vi "Encrypt.vi"(8 "error in (no error)":errorcluster, 10 "Arguments":string[](array[string]), 11 "Encryption in":refnum<class "Encryption.lvclass">) -> (0 "error out":errorcluster, 2 "Encrypted Arguments":string[](array[string]), 3 "Encryption out":refnum<class "Encryption.lvclass">)   [LabVIEW 2019, in "TSC Event Logger.lvlib" / "Encryption.lvclass"]
uses:
  Encryption.lvclass
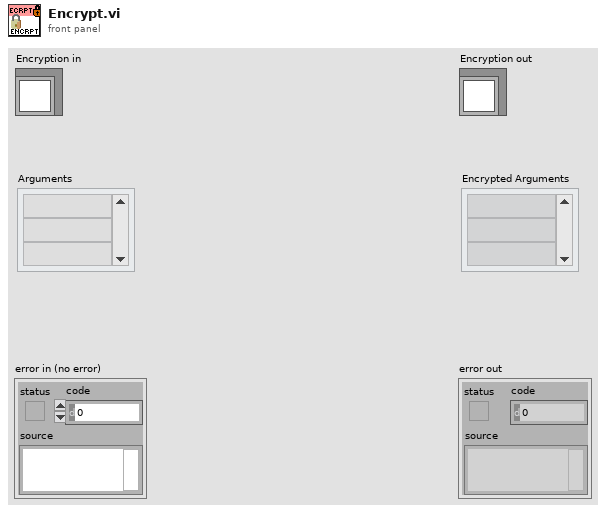
[diagram p1: front panel]
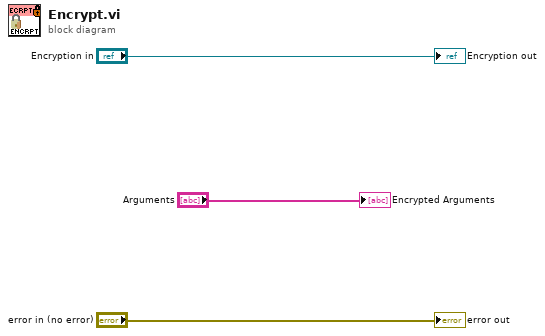
[diagram p0: block diagram]
diagram:
  "error out" <- "error in (no error)"
  "Encryption out" <- "Encryption in"
  "Encrypted Arguments" <- "Arguments"
